vi "Sub_sample_unique_pin_locations.vi"(9 "Modeling Parameters":T1, 10 "FEA Nodes":i32[](array[numeric]), 11 "Initial Pin Location":i32) -> (1 "Unique Samples":i32[](array[numeric]), 2 "Sample PDF":dbl[](array[numeric]), 3 "Standard Deviation":dbl)   [LabVIEW 2021]
uses:
  <vilib>/gmath/statdist.llb/Normal PDF.vi
  <vilib>/gmath/NI_Gmath.lvlib
panel:
  out "Waveform Graph":dbl[](graph)
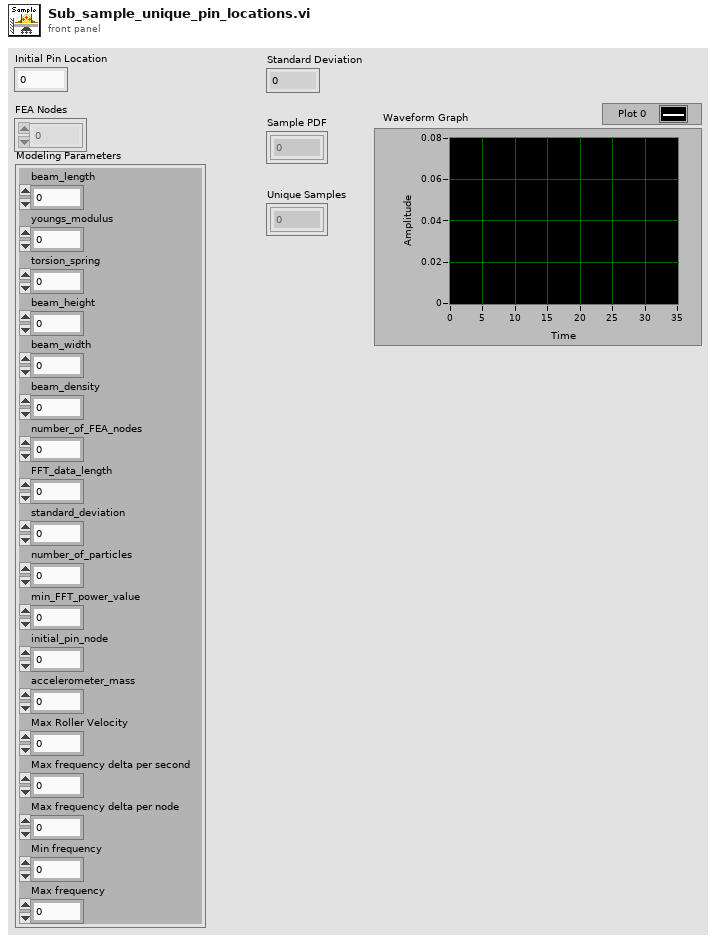
[diagram p1: front panel]
types:
  T1 = cluster{"beam_length":dbl, "youngs_modulus":dbl, "torsion_spring":dbl, "beam_height":dbl, "beam_width":dbl, "beam_density":dbl, "number_of_FEA_nodes":i32, "FFT_data_length":i32, "standard_deviation":dbl, "number_of_particles":i32, "min_FFT_power_value":dbl, "initial_pin_node":i32, "accelerometer_mass":dbl, "Max Roller Velocity":dbl, "Max frequency delta per second":dbl, "Max frequency delta per node":dbl, "Min frequency":dbl, "Max frequency":dbl}
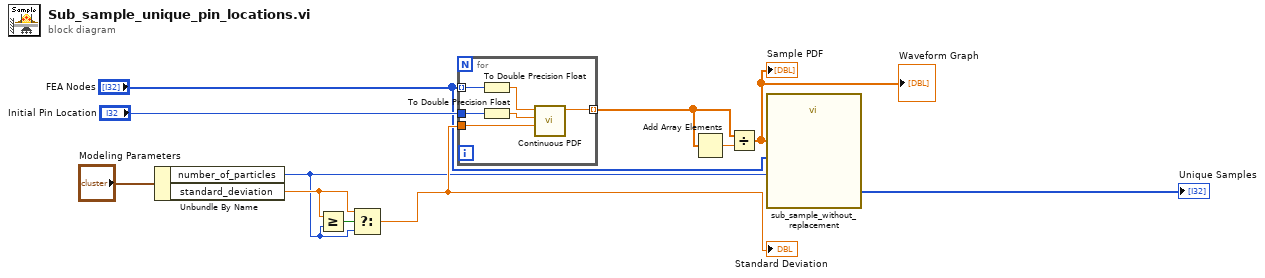
[diagram p0: block diagram]
diagram:
  n1 = Unbundle By Name("Modeling Parameters") -> ("number_of_particles"=w5:i32, "standard_deviation"=w7:dbl)
  n2 = Greater Or Equal?(x=w7, y=w5) -> (x >= y?=w8:bool)
  n3 = Select(t=w7, s=w8, f=w5) -> (s? t:f=w6:dbl)
  "Standard Deviation" <- w6
  n4 = for {
    tunnel: "FEA Nodes" -> [w14] mode=indexing
    tunnel: [w17] -> w9 mode=indexing
    tunnel: "Initial Pin Location" -> [w13]
    tunnel: w6 -> [w16]
    n5 = To Double Precision Float(number=w14) -> (double precision float=w15:dbl)
    n6 = To Double Precision Float(number=w13) -> (double precision float=w12:dbl)
    n7 = call-poly <vilib>:"Continuous PDF.vi"("std"=w16, "mean"=w12, "x"=w15) -> ("pdf(x)"=w17:dbl)  [unwired: 7 in, 1 out]
  }
  n8 = Add Array Elements(numeric array=w9) -> (sum=w11:dbl)
  n9 = Divide(x=w9, y=w11) -> (x/y=w2:dbl[])
  "Sample PDF" <- w2
  "Waveform Graph" <- w2
  n10 = call "sub_sample_without_replacement.vi"("number of unique samples"=w5, "probability"=w2, "List"="FEA Nodes") -> ("unique samples"=→"Unique Samples":i32[])  [unwired: 6 in, 2 out]
